vi "Cockpit UDP receiver function.vi"(11 "UDP connection ID":refnum<k16>) -> (0 "L3":sgl, 1 "L2":sgl, 2 "L1":sgl, 3 "UDP connection ID out":refnum<k16>, 4 "down_pedal":sgl format="%.2f", 5 "L4":sgl, 6 "right_pedal":bool, 7 "gripper":sgl, 8 "left_pedal":bool, 9 "up_pedal":bool)   [LabVIEW 2016]
panel:
  out "error IO":errorcluster
  out "length":i32
  out "data out":string
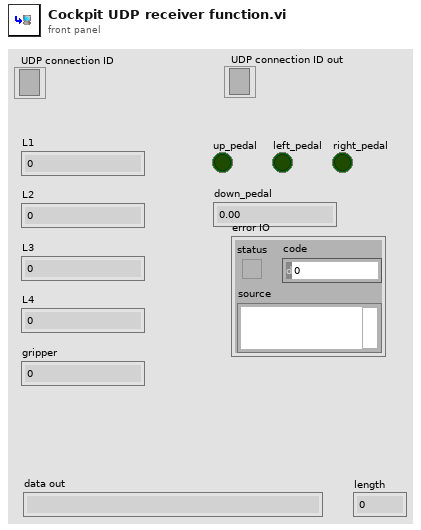
[diagram p1: front panel]
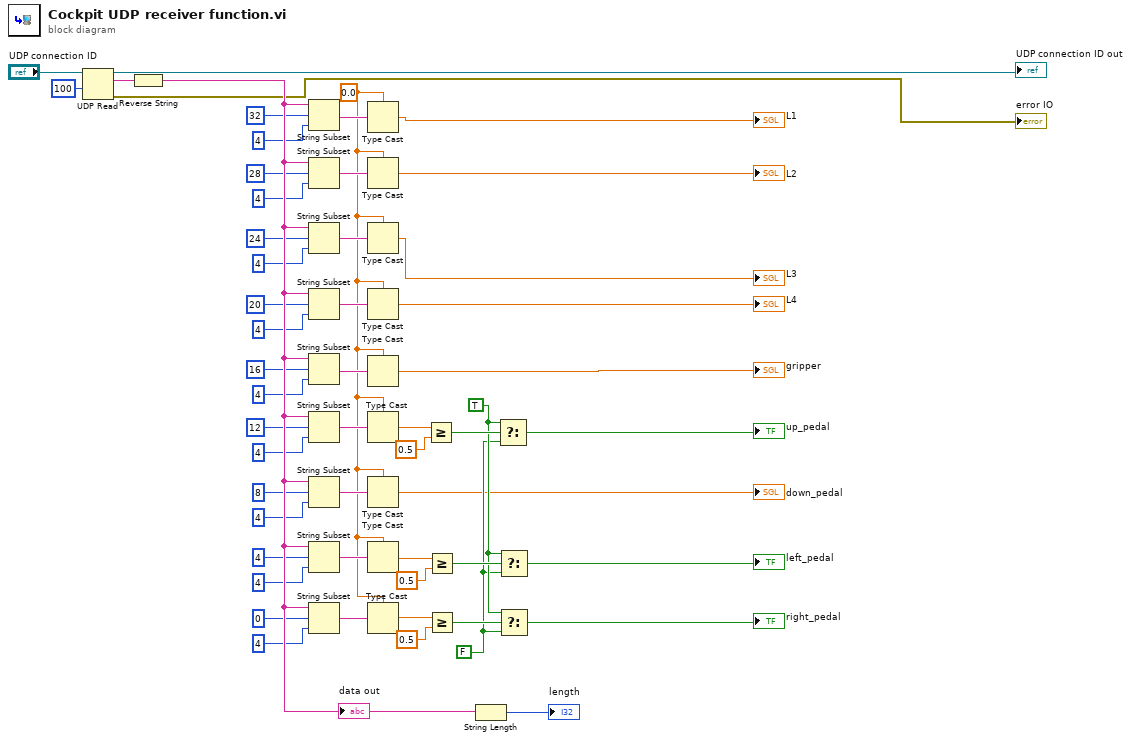
[diagram p0: block diagram]
diagram:
  w10 = FALSE
  w11 = TRUE
  w21 = sgl 0.0
  n1 = UDP Read(connection ID="UDP connection ID", timeout ms (25000)=100) -> (data out=w54:string, error out=→"error IO":errorcluster, 3:→"UDP connection ID out":refnum<k16>)  [unwired: 2 in, 2 out]
  n2 = Reverse String(1:w54) -> (0:w53:string)
  "data out" <- w53
  n3 = String Subset(string=w53, offset (0)=32, length (rest)=4 ("offset (0)")) -> (substring=w48:string)
  n4 = String Subset(string=w53, offset (0)=28, length (rest)=4 ("offset (0)")) -> (substring=w40:string)
  n5 = String Subset(string=w53, offset (0)=24, length (rest)=4 ("offset (0)")) -> (substring=w39:string)
  n6 = String Subset(string=w53, offset (0)=20, length (rest)=4 ("offset (0)")) -> (substring=w38:string)
  n7 = String Subset(string=w53, offset (0)=16, length (rest)=4 ("offset (0)")) -> (substring=w28:string)
  n8 = String Subset(string=w53, offset (0)=12, length (rest)=4 ("offset (0)")) -> (substring=w35:string)
  n9 = String Subset(string=w53, offset (0)=8, length (rest)=4 ("offset (0)")) -> (substring=w36:string)
  n10 = String Subset(string=w53, offset (0)=4, length (rest)=4 ("offset (0)")) -> (substring=w37:string)
  n11 = String Subset(string=w53, offset (0)=0, length (rest)=4 ("offset (0)")) -> (substring=w23:string)
  n12 = Type Cast(type=w21, x=w48) -> (*(type *) &x=→"L1":sgl)
  n13 = Type Cast(type=w21, x=w40) -> (*(type *) &x=→"L2":sgl)
  n14 = Type Cast(type=w21, x=w39) -> (*(type *) &x=→"L3":sgl)
  n15 = Type Cast(type=w21, x=w38) -> (*(type *) &x=→"L4":sgl)
  n16 = Type Cast(type=w21, x=w28) -> (*(type *) &x=→"gripper":sgl)
  n17 = Type Cast(type=w21, x=w35) -> (*(type *) &x=w18:sgl)
  n18 = Type Cast(type=w21, x=w36) -> (*(type *) &x=→"down_pedal":sgl)
  n19 = Type Cast(type=w21, x=w37) -> (*(type *) &x=w12:sgl)
  n20 = Type Cast(type=w21, x=w23) -> (*(type *) &x=w13:sgl)
  n21 = Greater Or Equal?(x=w18, y=sgl 0.5) -> (x >= y?=w20:bool)
  n22 = Greater Or Equal?(x=w12, y=sgl 0.5) -> (x >= y?=w16:bool)
  n23 = Greater Or Equal?(x=w13, y=sgl 0.5) -> (x >= y?=w15:bool)
  n24 = String Length(string=w53) -> (length=→"length":i32)
  n25 = Select(t=w11, s=w20, f=w10) -> (s? t:f=→"up_pedal":bool)
  n26 = Select(t=w11, s=w16, f=w10) -> (s? t:f=→"left_pedal":bool)
  n27 = Select(t=w11, s=w15, f=w10) -> (s? t:f=→"right_pedal":bool)
